vi "Lex Text-BeginSection.vi"(8 "Error In":errorcluster) -> (0 "Error Out":errorcluster)   [LabVIEW 2018, in "Tests.lvlib" / "Lexer.lvlib"]
uses:
  Lexer.lvlib
  <vilib>/addons/_JKI Toolkits/Caraya/classes/Test/Test.lvclass
  <vilib>/addons/_JKI Toolkits/Caraya/classes/Assert/Assert.lvclass
  src/Toolkit/Low-Level/Tokens/Token/Token.lvclass
  src/Toolkit/Low-Level/Tokens/Text/Text.lvclass
  Tests.lvlib
  src/Toolkit/Low-Level/Tokens/BeginSection/BeginSection.lvclass
  src/Toolkit/Low-Level/Support/Lex String.vi
  D:/Users/cfield/Code/Field R&D Services/Labstache/src/Toolkit/Low-Level/Tokens/Contentable/Contentable.lvclass
  D:/Users/cfield/Code/Field R&D Services/Labstache/src/Toolkit/Low-Level/Tokens/Token/Token.lvclass
  D:/Users/cfield/Code/Field R&D Services/Labstache/src/Toolkit/Low-Level/Tokens/Keyable/Keyable.lvclass
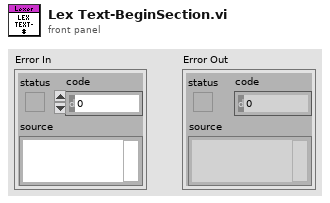
[diagram p1: front panel]
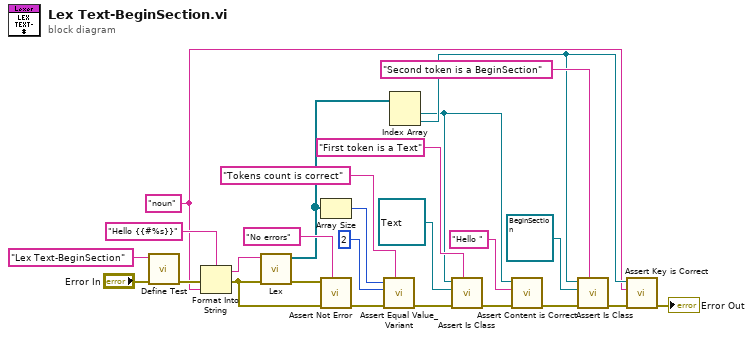
[diagram p0: block diagram]
diagram:
  w6 = "noun" ("String")
  n1 = call <vilib>:"Define Test.vi"("error in (no error)"="Error In", "Label (VI Title)"="Lex Text-BeginSection") -> ("error out"=w23:errorcluster)  [unwired: 9 in]
  n2 = Format Into String(format string="Hello {{#%s}}", error in=w23, w6) -> (resulting string=w2:string, error out=w1:errorcluster)  [unwired: 1 in]
  n3 = call-poly "Lex.vi"("Error In"=w1, "Input"=w2) -> ("Error Out"=w24:errorcluster, "Tokens"=w16:refnum<class "Token.lvclass">[])  [unwired: 8 in]
  n4 = Array Size(array=w16) -> (size(s)=w19:i32)
  n5 = call <vilib>:"Assert Not Error.vi"("Label"="No errors", "error in (no error)"=w1, "Not Error?"=w24) -> ("error out"=w21:errorcluster)  [unwired: 8 in]
  n6 = call <vilib>:"Assert Equal Value_Variant.vi"("Label"="Tokens count is correct", "error in (no error)"=w21, "Y"=2 ("size(s)"), "X"=w19) -> ("error out"=w17:errorcluster)  [unwired: 7 in]
  n7 = Index Array(array=w16) -> (element #1=w4:refnum<class "Token.lvclass">, element #2=w8:refnum<class "Token.lvclass">)  [unwired: 2 in]
  n8 = call "Assert Is Class.vi"("Label"="First token is a Text", "Error In"=w17, "Expected"=refnum<class "Text.lvclass"> refnum ("Mustache.lvlib:Tokens.lvlib:Text.lvclass"), "Actual"=w4) -> ("Error Out"=w14:errorcluster)  [unwired: 7 in]
  n9 = call "Assert Content is Correct.vi"("Error In"=w14, "Expected"="Hello ", "Token"=w4) -> ("Error Out"=w13:errorcluster)  [unwired: 8 in]
  n10 = call "Assert Is Class.vi"("Label"="Second token is a BeginSection", "Error In"=w13, "Expected"=refnum<class "BeginSection.lvclass"> refnum ("Mustache.lvlib:Tokens.lvlib:BeginSection.lvclass"), "Actual"=w8) -> ("Error Out"=w7:errorcluster)  [unwired: 7 in]
  n11 = call "Assert Key is Correct.vi"("Error In"=w7, "Expected"=w6, "Token"=w8) -> ("Error Out"=→"Error Out":errorcluster)  [unwired: 8 in]
